vi "Check mac in range.vi"(6 "MAC range end":string, 8 "error in (no error)":errorcluster, 9 "MAC range start":string, 10 "MAC prefix":string, 11 "MAC":string) -> (0 "error out":errorcluster, 3 "In Range?":bool)   [LabVIEW 2013]
panel:
  out "MAC max offset":u32
  out "MAC min offset":u32
  out "MAC offset num":u32
  out "MAC range end offset":string
  out "MAC range start offset":string
  out "MAC offset":string
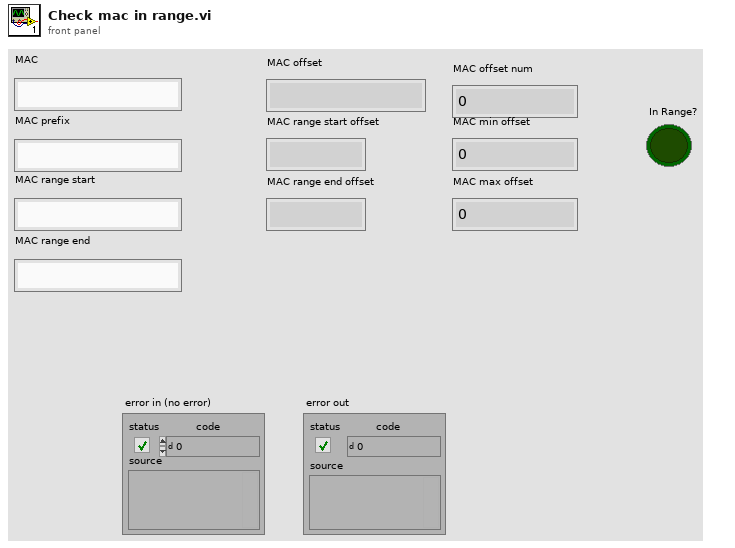
[diagram p1: front panel]
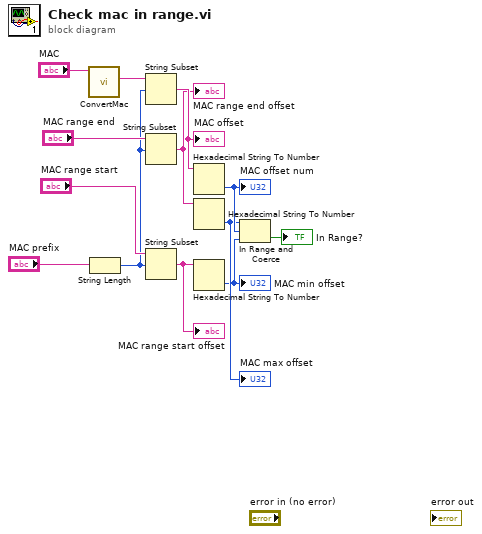
[diagram p0: block diagram]
diagram:
  n1 = call "ConvertMac.vi"("Mac (with or without semicolons)"="MAC") -> ("Mac without semi"=w11:string)  [unwired: 8 in, 2 out]
  n2 = String Length(string="MAC prefix") -> (length=w8:i32)
  n3 = String Subset(string=w11, offset (0)=w8) -> (substring=w7:string)  [unwired: 1 in]
  "MAC offset" <- w7
  n4 = String Subset(string="MAC range end", offset (0)=w8) -> (substring=w5:string)  [unwired: 1 in]
  "MAC range end offset" <- w5
  n5 = String Subset(string="MAC range start", offset (0)=w8) -> (substring=w6:string)  [unwired: 1 in]
  "MAC range start offset" <- w6
  n6 = Hexadecimal String To Number(string=w7) -> (number=w4:u32)  [unwired: 2 in, 1 out]
  "MAC offset num" <- w4
  n7 = Hexadecimal String To Number(string=w5) -> (number=w3:u32)  [unwired: 2 in, 1 out]
  "MAC max offset" <- w3
  n8 = Hexadecimal String To Number(string=w6) -> (number=w2:u32)  [unwired: 2 in, 1 out]
  "MAC min offset" <- w2
  n9 = In Range and Coerce(upper limit=w3, x=w4, lower limit=w2) -> (In Range?=→"In Range?":bool)  [unwired: 1 out]
